vi "Create Serial Master.vi"(4 "flow control (none)":u16(ring) items=["None", "XON/XOFF", "RTS/CTS", "XON/XOFF & RTS/CTS", "DTR/DSR", "XON/XOFF & DTR/DSR"], 5 "serial type":enum16{"RTU", "ASCII"}(ring), 6 "parity (even)":u16(ring)=2 items=["None", "Odd", "Even", "Mark", "Space"], 7 "unit ID":u8=1, 8 "error in":errorcluster, 10 "baud rate":u32=9600, 11 "VISA resource name":refnum<visa-resource-name>) -> (0 "error out":errorcluster, 3 "serial master instance":refnum<class "Modbus Master.lvclass">)   [LabVIEW 2015, in "Modbus Library.lvlib" / "API Main.lvlib"]
doc: "Creates a standard serial master. The transmission data unit used by the device is defined by the <B>serial type</B> input."
uses:
  API Main.lvlib
  Master/Modbus Master.lvclass
  Master Function Definition/Master Function Definition.lvclass
  Network Protocol/Network Master/Serial/Serial Master.lvclass
  Transmission Data Unit/RTU/RTU Data Unit.lvclass
  Transmission Data Unit/ASCII/ASCII Data Unit.lvclass
  Modbus API.lvclass
  Transmission Data Unit/Transmission Data Unit.lvclass
panel:
  # "disable parity disallowed by mbspec"
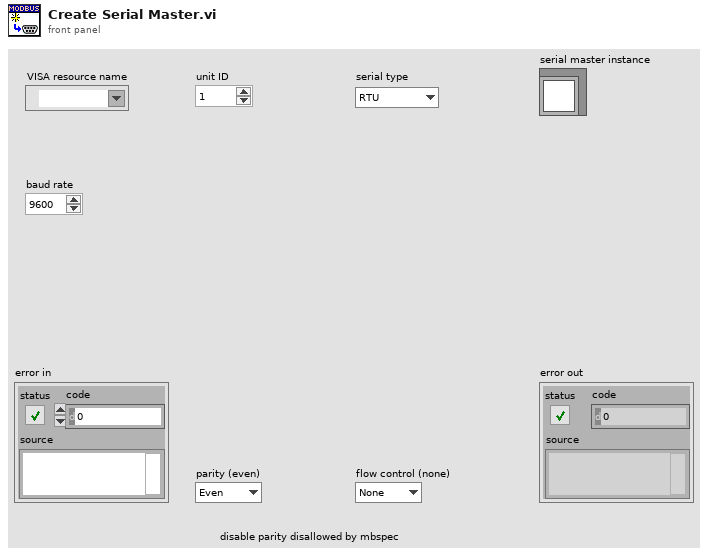
[diagram p1: front panel]
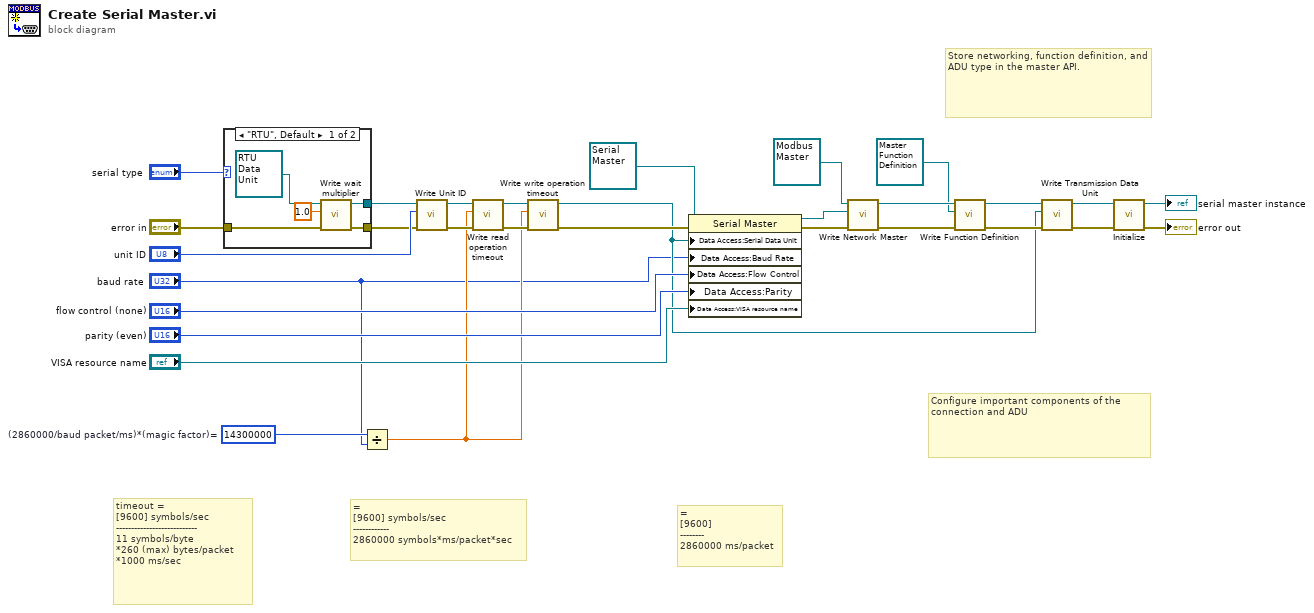
[diagram p0: block diagram]
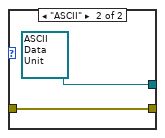
[diagram p2: hidden frame]
diagram:
  w11 = u32 14300000  # (2860000/baud packet/ms)*(magic factor)=
  # "=\n[9600]\n--------\n2860000 ms/packet"
  # "=\n[9600] symbols/sec\n------------\n2860000 symbols*ms/packet*sec"
  # "timeout =\n[9600] symbols/sec\n---------------------------\n11 symbols/byte\n*260 (max) bytes/packet\n*1000 ms/sec"
  # "Configure important components of the connection and ADU"
  # "Store networking, function definition, and ADU type in the master API."
  n1 = case shown="\"RTU\", Default" "serial type" {
    tunnel: [w35 refnum<class "ASCII Data Unit.lvclass"> refnum ("ASCII Data Unit")] -> w13
    tunnel: "error in" -> [w33 w36]
    tunnel: [w34 w36] -> w1
    frame "RTU", Default {
      n2 = call "Write wait multiplier.vi"("error in (no error)"=w33, "wait multiplier"=sgl 1.0, "RTU Data Unit in"=refnum<class "RTU Data Unit.lvclass"> refnum ("RTU Data Unit")) -> ("error out"=w34:errorcluster, "RTU Data Unit out"=w35:refnum<class "RTU Data Unit.lvclass">)  [unwired: 7 in]
    }
    frame "ASCII" {
    }
  }
  n3 = Divide(x=w11, y="baud rate") -> (x/y=w4:dbl)
  n4 = call "Write Unit ID.vi"("error in"=w1, "unit ID"="unit ID", "transmission data unit in"=w13) -> ("error out"=w8:errorcluster, "transmission data unit out"=w9:refnum<class "Serial Data Unit.lvclass">)  [unwired: 7 in]
  n5 = call "Write read operation timeout.vi"("error in (no error)"=w8, "read operation timeout"=w4, "transmission data unit in"=w9) -> ("error out"=w7:errorcluster, "transmission data unit out"=w10:refnum<class "Serial Data Unit.lvclass">)  [unwired: 7 in]
  n6 = call "Write write operation timeout.vi"("error in (no error)"=w7, "write operation timeout"=w4, "transmission data unit in"=w10) -> ("error out"=w6:errorcluster, "transmission data unit out"=w5:refnum<class "Serial Data Unit.lvclass">)  [unwired: 7 in]
  n7 = property class="Serial Master"(reference=refnum<class "Serial Master.lvclass"> refnum ("Serial Master"), error in=w6, "Data Access:Serial Data Unit"=w5, "Data Access:Baud Rate"="baud rate", "Data Access:Flow Control"="flow control (none)", "Data Access:Parity"="parity (even)", "Data Access:VISA resource name"="VISA resource name") -> (reference out=w14:refnum<class "Serial Master.lvclass">, error out=w23:errorcluster)
  n8 = call "Write Network Master.vi"("error in"=w23, "network master"=w14, "Modbus master in"=refnum<class "Modbus Master.lvclass"> refnum ("Modbus Master")) -> ("error out"=w16:errorcluster, "Modbus master out"=w21:refnum<class "Modbus Master.lvclass">)  [unwired: 7 in]
  n9 = call "Write Function Definition.vi"("error in"=w16, "master function definition"=refnum<class "Master Function Definition.lvclass"> refnum ("Master Function Definition"), "Modbus master in"=w21) -> ("error out"=w17:errorcluster, "Modbus master out"=w20:refnum<class "Modbus Master.lvclass">)  [unwired: 7 in]
  n10 = call "Write Transmission Data Unit.vi"("error in"=w17, "transmission data unit"=w5, "Modbus instance in"=w20) -> ("error out"=w18:errorcluster, "Modbus instance out"=w19:refnum<class "Modbus Master.lvclass">)  [unwired: 7 in]
  n11 = call-dynamic "Initialize.vi"("error in"=w18, "Modbus master in"=w19) -> ("error out"=→"error out":errorcluster, "Modbus master out"=→"serial master instance":refnum<class "Modbus Master.lvclass">)  [unwired: 8 in]
